vi "subExportContainerContent.vi"(6 "CodeSchema":string, 8 "error in (no error)":errorcluster, 9 "Expand?":bool, 11 "ILabVIEWItem in":refnum<class "ILabVIEWItem.lvclass">) -> (0 "error out":errorcluster, 1 "Links":T1, 2 "Nodes":T1, 3 "ILabVIEWItem out":refnum<class "ILabVIEWItem.lvclass">)   [LabVIEW 2020, in "DefaultExtensions.lvlib" / "CGrapherDGML.lvclass"]
uses:
  CGrapherDGML.lvclass
  obj/Addons/LabVIEWObjectInterfaces.lvlibp/LabVIEWObjectInterfaces/ILabVIEWItem/ILabVIEWItem.lvclass
  obj/Addons/LabVIEWItem.lvlibp/LabVIEWItem/CLabVIEWItem/ConnectionSet.ctl
  02eefc4a-eede-484c-8d24-8de4f53580c2.vi
  obj/Addons/LabVIEWItem.lvlibp/LabVIEWItem/CLabVIEWItem/CLabVIEWItem.lvclass
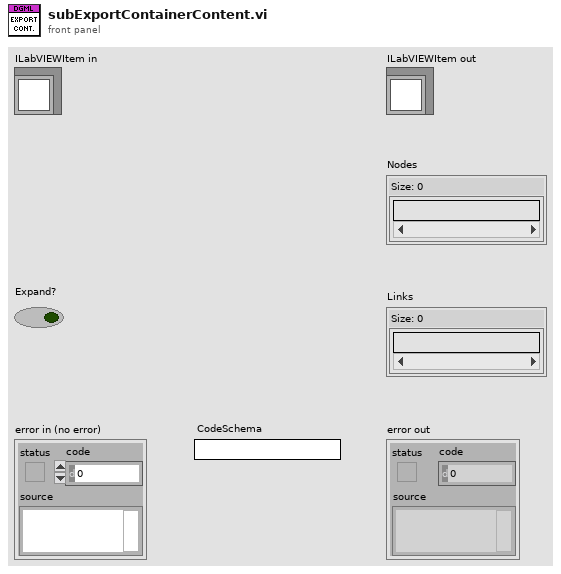
[diagram p1: front panel]
types:
  T1 = typedef "LabVIEWItem.lvlibp/CLabVIEWItem.lvclass/ConnectionSet.ctl" = set{string}
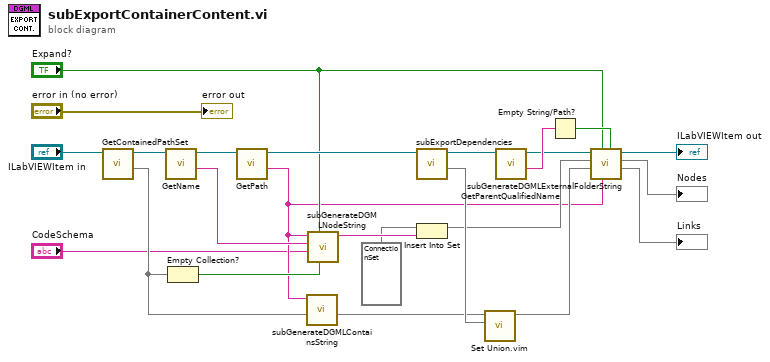
[diagram p0: block diagram]
diagram:
  n1 = call-dynamic "GetContainedPathSet.vi"("ILabVIEWItem in"="ILabVIEWItem in") -> ("Contained"=w6:set{string}, "ILabVIEWItem out"=w2:refnum<class "ILabVIEWItem.lvclass">)  [unwired: 8 in, 1 out]
  n2 = call-dynamic "GetName.vi"("ILabVIEWItem in"=w2) -> ("Name"=w20:string, "ILabVIEWItem out"=w24:refnum<class "ILabVIEWItem.lvclass">)  [unwired: 8 in, 1 out]
  n3 = Empty Collection?(1:w6) -> (0:w19:bool)
  n4 = call-dynamic "GetPath.vi"("ILabVIEWItem in"=w24) -> ("Path"=w10:string, "ILabVIEWItem out"=w22:refnum<class "ILabVIEWItem.lvclass">)  [unwired: 8 in, 1 out]
  n5 = call "subGenerateDGMLContainsString.vi"("Contained"=w6, "Source"=w10) -> ("Links"=w17:T1)  [unwired: 9 in]
  n6 = call "subGenerateDGMLNodeString.vi"("Container empty?"=w19, "Expand?"="Expand?", "Code schema"="CodeSchema", "Label"=w20, "Id"=w10) -> ("Node string"=w18:string)  [unwired: 6 in]
  n7 = call "subExportDependencies.vi"("ILabVIEWItem in"=w22) -> ("Links"=w21:T1, "ILabVIEWItem out"=w16:refnum<class "ILabVIEWItem.lvclass">)  [unwired: 8 in, 1 out]
  n8 = Insert Into Set(10:w18, 11:T1 {} ("Links")) -> (3:w14:T1)  [unwired: 1 out]
  n9 = call "Set Union.vim"("set 2"=w21, "set 1"=w17) -> ("union"=w11:T1)  [unwired: 9 in]
  n10 = call-dynamic "GetParentQualifiedName.vi"("ILabVIEWItem in"=w16) -> ("Name"=w15:string, "ILabVIEWItem out"=w5:refnum<class "ILabVIEWItem.lvclass">)  [unwired: 8 in, 1 out]
  n11 = Empty String/Path?(string/path=w15) -> (empty?=w13:bool)
  n12 = call "subGenerateDGMLExternalFolderString.vi"("Apply? (T)"=w13, "Path in"=w10, "Expand?"="Expand?", "Links in"=w11, "Nodes in"=w14, "ILabVIEWItem in"=w5) -> ("Links"=→"Links":T1, "Nodes"=→"Nodes":T1, "ILabVIEWItem out"=→"ILabVIEWItem out":refnum<class "ILabVIEWItem.lvclass">)  [unwired: 2 in, 1 out]
  "error out" <- "error in (no error)"
